vi "Insert View.vi"(8 "error in (no error)":errorcluster, 9 "Insertion Request Time":timestamp, 10 "Protected Subpanel":T1, 11 "MultiSubscriber In":refnum<class "MultiSubscriber.lvclass">) -> (0 "error out":errorcluster, 3 "MultiSubscriber Out":refnum<class "MultiSubscriber.lvclass">)   [LabVIEW 2018, in "TestViewables.lvlib" / "MultiSubscriber.lvclass"]
doc: "<License>\nCopyright © 2017 Composed Systems, LLC | All rights reserved\nwww.composed.io\n\nAuthor: Ethan Stern <ethan.stern@composed.io>\n\nThis software is provided \"AS IS\" WITHOUT WARRANTIES, either express or implied, AND IS FOR EDUCATIONAL PURPOSES ONLY.\n</License>"
uses:
  MultiSubscriber.lvclass
  modules/mva-viewable/Source/IViewable/ProtectedSubpanel/Protected Subpanel Reference.ctl
  modules/mva-viewable/Source/IViewable/ProtectedSubpanel/ProtectedSubpanel.lvclass
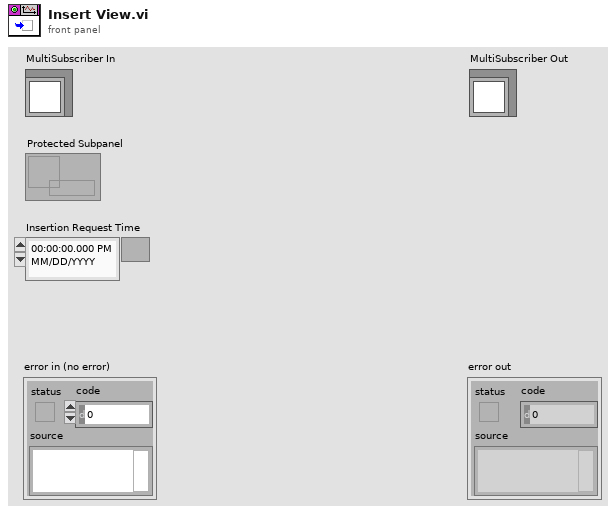
[diagram p1: front panel]
types:
  T1 = typedef "MVA Framework.lvlib/IViewable.lvlib/ProtectedSubpanel.lvclass/Protected Subpanel Reference.ctl" = refnum<data-value>
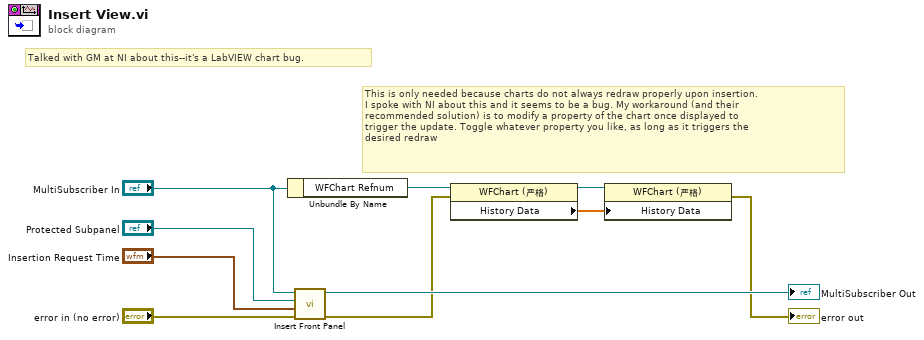
[diagram p0: block diagram]
diagram:
  # "This is only needed because charts do not always redraw properly upon insertion.\nI spoke with NI about this and it seems to be a bug. My workaround (and their\nrecommended solution) is to modify a property of the chart once displayed to\ntrigger the update. Toggle whatever property you like, as long as it triggers the\ndesired redraw"
  # "Talked with GM at NI about this--it's a LabVIEW chart bug."
  n1 = Unbundle By Name("MultiSubscriber In") -> ("WFChart Refnum"=w3:refnum<vi>)
  n2 = call-dynamic "Insert Front Panel.vi"("error in (no error)"="error in (no error)", "Insertion Request Time"="Insertion Request Time", "Protected Subpanel"="Protected Subpanel", "IViewable in"="MultiSubscriber In") -> ("error out"=w2:errorcluster, "IViewable out"=→"MultiSubscriber Out":refnum<class "MultiSubscriber.lvclass">)  [unwired: 6 in]
  n3 = property class="WFChart (严格)"(reference=w3, error in=w2) -> (reference out=w6:refnum<vi>, "History Data"=w5:dbl[])  [unwired: 1 out]
  n4 = property class="WFChart (严格)"(reference=w6, "History Data"=w5) -> (error out=→"error out":errorcluster)  [unwired: 1 in, 1 out]
